vi "Demo- Create and Update Feature Studio in default document.vi"() -> ()   [LabVIEW 2019]
panel:
  in  "FeatureScript":string
  in  "New Feature Studio Name":string="demo"
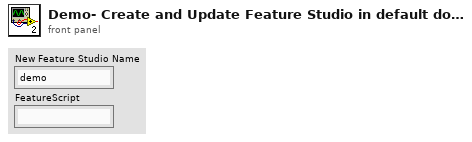
[diagram p1: front panel]
types:
  T1 = cluster{"Date":string, "On-Nonce":string, "ctype":string, "path":string, "method":string, "Authorization":string, "Accept":string, "User-Agent":string, "Content-Type":string, "secret_key":string, "access_key":string, "stack":string, "payload":string, "headers":string[], "eid":string, "wid":string, "did":string, "name":string}
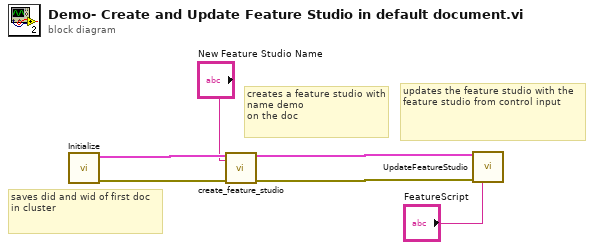
[diagram p0: block diagram]
diagram:
  # "updates the feature studio with the feature studio from control input"
  # "creates a feature studio with name demo\non the doc"
  # "saves did and wid of first doc in cluster"
  n1 = call "Initialize.vi"() -> ("error out"=w4:errorcluster, "Device Out"=w6:T1)  [unwired: 9 in, 1 out]
  n2 = call "create_feature_studio.vi"("Device In"=w6, "New Feature Studio Name"="New Feature Studio Name", "error in"=w4) -> ("Device Out"=w3:T1, "error out"=w2:errorcluster)  [unwired: 10 in, 1 out]
  n3 = call "UpdateFeatureStudio.vi"("Device In"=w3, "error in"=w2, "FeatureScript"="FeatureScript") -> ()  [unwired: 10 in, 3 out]
